vi "set_logging.vi"(8 "error in (no error)":errorcluster, 10 "system.logging.lvclass":refnum<class "system.logging.lvclass">, 11 "system in":refnum<class "system.lvclass">) -> (0 "error out":errorcluster, 3 "system out":refnum<class "system.lvclass">)   [LabVIEW 2021, in "system.lvclass"]
uses:
  system.lvclass
  system.lvclass/system.ctl
  system.logging/system.logging.lvclass
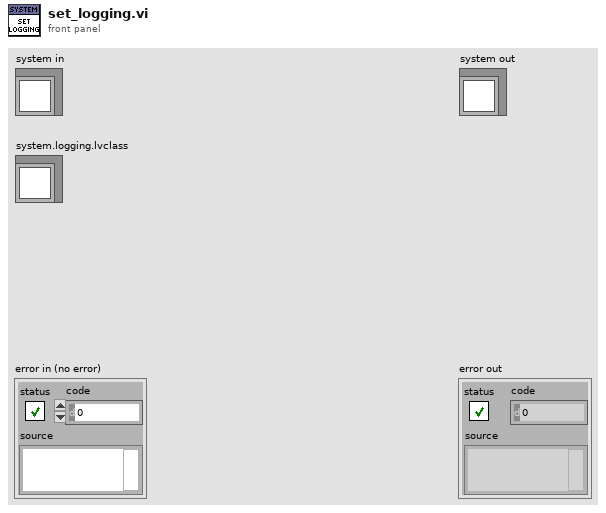
[diagram p1: front panel]
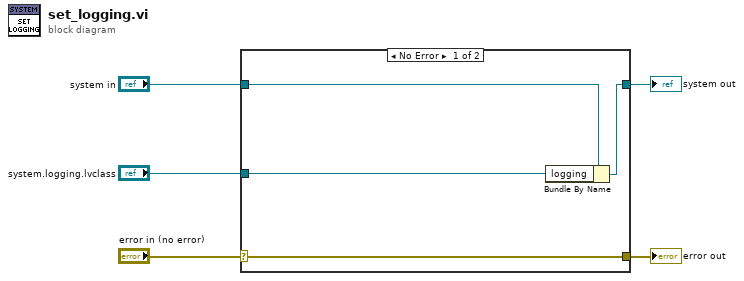
[diagram p0: block diagram]
diagram:
  n1 = case shown="No Error" "error in (no error)" {
    selector: "error in (no error)" -> [w9 w10]
    tunnel: [w9 w10] -> w4
    tunnel: [w7 w11] -> w2
    tunnel: "system in" -> [w8 w11]
    tunnel: "system.logging.lvclass" -> [w6 _]
    frame No Error {
      n2 = Bundle By Name(cluster=w8, "logging"=w6) -> (w7:refnum<class "system.lvclass">)
    }
    frame Error {
    }
  }
  "error out" <- w4
  "system out" <- w2
